vi "Handle.vi"(10 "log record":T1 {"timestamp" format="%<%x %.3X>T"}, 11 "test handler in":refnum<class "Test Handler.lvclass">) -> (0 "writer error":errorcluster, 1 "formatter error":errorcluster, 3 "test handler out":refnum<class "Test Handler.lvclass">)   [LabVIEW 2018, in "Test Handler.lvclass"]
uses:
  Test Handler.lvclass
  src/api/logger_class/Log Record.ctl
  src/api/logger_class/Internal Log Levels.ctl
  Test Handler.lvclass/Test Handler.ctl
  <vilib>/Utility/config.llb/Read Key (Boolean).vi
  <vilib>/Utility/error.llb/Error Cluster From Error Code.vi
  <vilib>/ErrorRing/Error Ring.xnode
  src/api/extension/formatting_handler_interface/Formatting Handler.lvclass
  <vilib>/Utility/config.llb/NI_LVConfig.lvlib
  dependencies/Utilities/Utilities.lvlib
  src/api/logger_class/Logger.lvclass
panel:
  # "Connector Pane"
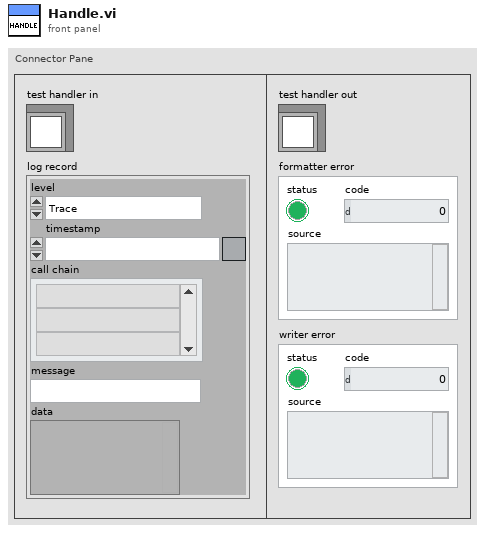
[diagram p1: front panel]
types:
  T1 = typedef "GLog.lvlib/Logger.lvclass/Log Record.ctl" = cluster{"level":T2, "timestamp":timestamp, "call chain":string[], "message":string, "data":variant}
  T2 = typedef "GLog.lvlib/Logger.lvclass/Internal Log Levels.ctl" = enum16{"Trace", "Debug", "Info", "Warning", "Error", "Critical", "Internal"}
  T3 = typedef "NI_LVConfig.lvlib/Config Data RefNum.ctl" = refnum<k1>
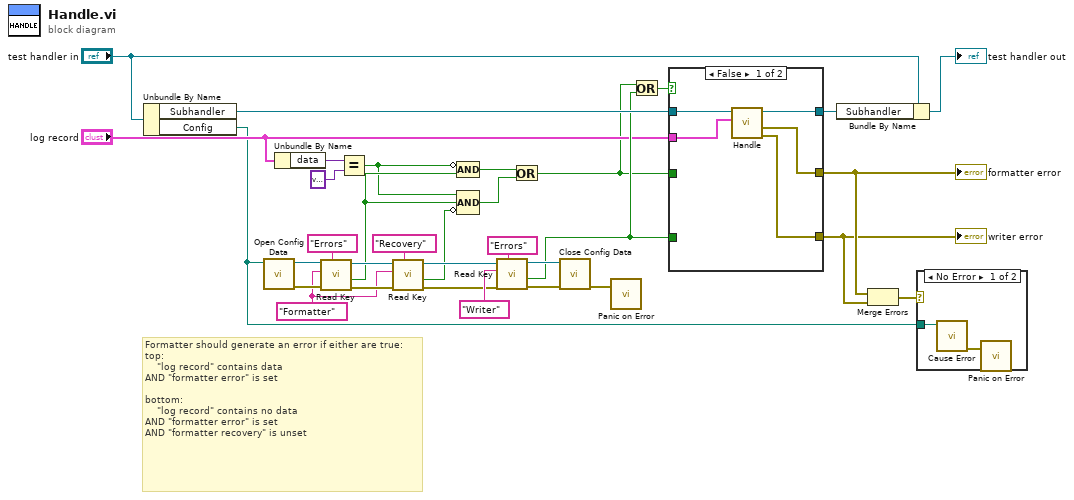
[diagram p0: block diagram]
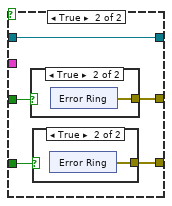
[diagram p3: hidden frame]
diagram:
  w8 = "Formatter" ("key")
  # "Formatter should generate an error if either are true:\ntop:\n    \"log record\" contains data\nAND \"formatter error\" is set\n\nbottom:\n    \"log record\" contains no data\nAND \"formatter error\" is set\nAND \"formatter recovery\" is unset"
  n1 = Unbundle By Name("test handler in") -> ("Subhandler"=w33:refnum<class "Formatting Handler.lvclass">, "Config"=w14:path)
  n2 = call <vilib>:"Open Config Data.vi"("configuration file path"=w14) -> ("error out"=w27:errorcluster, "refnum"=w28:T3)  [unwired: 8 in, 1 out]
  n3 = Unbundle By Name("log record") -> ("data"=w19:variant)
  n4 = call-poly <vilib>:"Read Key.vi"("section"="Errors" ("key"), "error in (no error)"=w27, "key"=w8, "refnum"=w28) -> ("error out"=w26:errorcluster, "value"=w7:bool, "refnum out"=w11:T3)  [unwired: 4 in, 1 out]
  n5 = Equal?(x=w19, y=variant) -> (x = y?=w2:bool)
  n6 = call-poly <vilib>:"Read Key.vi"("section"="Recovery" ("key"), "error in (no error)"=w26, "key"=w8, "refnum"=w11) -> ("error out"=w12:errorcluster, "value"=w6:bool, "refnum out"=w10:T3)  [unwired: 4 in, 1 out]
  n7 = Compound Arithmetic op=AND(invert w2, w7) -> (w4:bool)
  n8 = Compound Arithmetic op=AND(w2, w7, invert w6) -> (w5:bool)
  n9 = call-poly <vilib>:"Read Key.vi"("section"="Errors" ("key"), "error in (no error)"=w12, "key"="Writer", "refnum"=w10) -> ("error out"=w24:errorcluster, "value"=w21:bool, "refnum out"=w25:T3)  [unwired: 4 in, 1 out]
  n10 = Or(x=w4, y=w5) -> (x .or. y?=w3:bool)
  n11 = call <vilib>:"Close Config Data.vi"("error in (no error)"=w24, "refnum"=w25) -> ("error out"=w20:errorcluster)  [unwired: 8 in, 1 out]
  n12 = call "Panic on Error.vi"("error in (no error)"=w20) -> ()  [unwired: 3 in]
  n13 = Or(x=w3, y=w21) -> (x .or. y?=w29:bool)
  n14 = case shown="False" w29 {
    tunnel: [w38 w40] -> w15
    tunnel: [w37 w42] -> w16
    tunnel: "log record" -> [w36 _]
    tunnel: w33 -> [w35 w43]
    tunnel: [w34 w43] -> w31
    tunnel: w3 -> [_ w41]
    tunnel: w21 -> [_ w39]
    frame False {
      n15 = call-dynamic "Handle.vi"("log record"=w36, "handler in"=w35) -> ("writer error"=w38:errorcluster, "formatter error"=w37:errorcluster, "handler out"=w34:refnum<class "Formatting Handler.lvclass">)  [unwired: 7 in]
    }
    frame True {
      n16 = case shown="True" w41 {
        tunnel: [_ w44] -> w42
        frame False {
        }
        frame True {
          n17 = xnode "Error Ring"() -> ("error out"=w44:errorcluster)
        }
      }
      n18 = case shown="True" w39 {
        tunnel: [_ w50] -> w40
        frame False {
        }
        frame True {
          n19 = xnode "Error Ring"() -> ("error out"=w50:errorcluster)
        }
      }
    }
  }
  "writer error" <- w15
  "formatter error" <- w16
  n20 = Bundle By Name(cluster="test handler in", "Subhandler"=w31) -> (→"test handler out":refnum<class "Test Handler.lvclass">)
  n21 = Merge Errors(w16, w15) -> (w13:errorcluster)
  n22 = case shown="No Error" w13 {
    tunnel: w14 -> [w57 _]
    frame No Error {
      n23 = call "Cause Error.vi"("ini file path"=w57) -> ("error out"=w56:errorcluster)  [unwired: 9 in, 1 out]
      n24 = call "Panic on Error.vi"("error in (no error)"=w56) -> ()  [unwired: 3 in]
    }
    frame Error {
    }
  }
